vi "Do Action.vi"(7 "Self Enqueuer":refnum<class "Message Enqueuer.lvclass">, 8 "error in (no error)":errorcluster, 11 "Change Column Header in":refnum<class "Change Column Header.lvclass">) -> (0 "error out":errorcluster)   [LabVIEW 2016, in "Assert API Components.lvlib" / "Assert Display.lvlib" / "Main Display.lvlib" / "Change Column Header.lvclass"]
uses:
  Change Column Header.lvclass
  <vilib>/ActorFramework/Message Enqueuer/Message Enqueuer.lvclass
  Change Column Header.lvclass/Change Column Header.ctl
  Main Display Messages/Set Column Header Msg/Set Column Header Msg.lvclass/Set Column Header Msg.ctl
  <vilib>/ActorFramework/Message Enqueuer/Message Enqueuer.lvclass/Message Enqueuer.ctl
  <vilib>/ActorFramework/Message Enqueuer/Enqueue.vi
  Main Display Messages/Set Column Header Msg/Set Column Header Msg.lvclass
  C:/Program Files (x86)/National Instruments/LabVIEW 2016/vi.lib/ActorFramework/Message/Message.lvclass
  <vilib>/Utility/LVClass/Get LV Class Name.vi
  <resource>/AFDebug/Generate Trace for Message.vi
  <vilib>/ActorFramework/Message Priority Queue/Priority Enqueue.vi
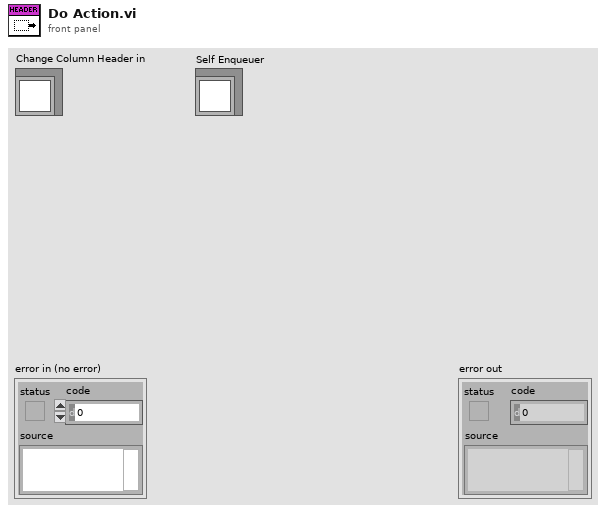
[diagram p1: front panel]
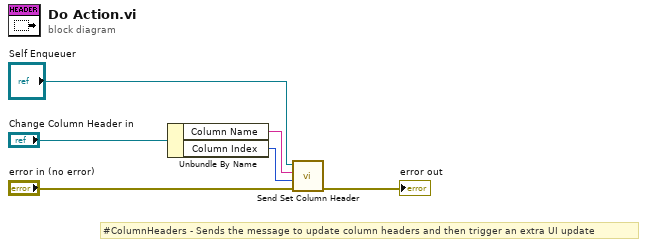
[diagram p0: block diagram]
diagram:
  # "#ColumnHeaders - Sends the message to update column headers and then trigger an extra UI update"
  n1 = Unbundle By Name("Change Column Header in") -> ("Column Name"=w5:string, "Column Index"=w4:i32)
  n2 = call "Send Set Column Header.vi"("error in (no error)"="error in (no error)", "Column Index"=w4, "Column Name"=w5, "Message Enqueuer"="Self Enqueuer") -> ("error out"=→"error out":errorcluster)  [unwired: 6 in, 1 out]
